vi "Read Acquisition Interface.vi"(8 "error in (no error)":errorcluster, 11 "Control_interface in":refnum<class "Control_interface.lvclass">) -> (0 "error out":errorcluster, 2 "Acquisition Interface":T1={"Sample Rate"=6000000000.0, "Clock mode"=enum."Internal", "Mode"=0, "Depth"=816000.0, "Segment Size"=816000.0, "Trigger Timeout"=-1.0, "Trigger Holdoff"=0.0, "Trigger Delay"=0.0} {"Segment Size" min=160.0 step=160.0; "Trigger Holdoff" min=0.0 step=160.0; "Trigger Delay" min=0.0 step=160.0; "Depth" min=160.0 step=160.0; "Mode" items=["Single", "Dual", "Quad", "Octal"]}, 3 "Control_interface out":refnum<class "Control_interface.lvclass">)   [LabVIEW 2015, in "Control_interface.lvclass"]
uses:
  Control_interface.lvclass
  Control_interface.lvclass/Control_interface.ctl
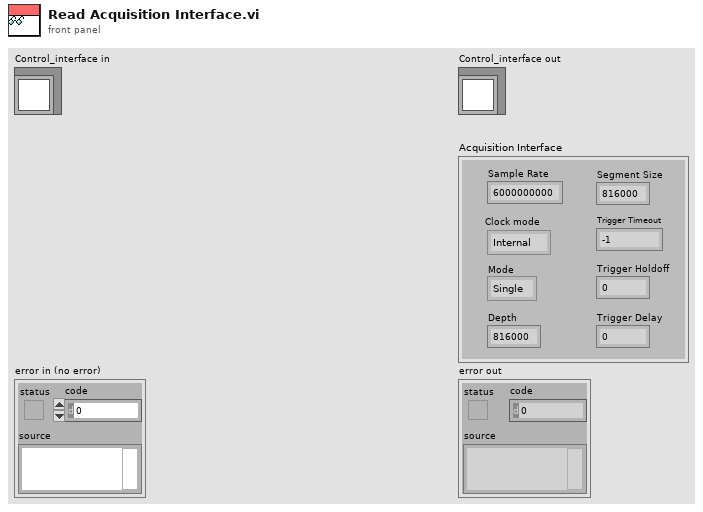
[diagram p1: front panel]
types:
  T1 = cluster{"Sample Rate":dbl, "Clock mode":enum16{"Internal", "External", "Reference"}, "Mode":u16, "Depth":dbl, "Segment Size":dbl, "Trigger Timeout":dbl, "Trigger Holdoff":dbl, "Trigger Delay":dbl}
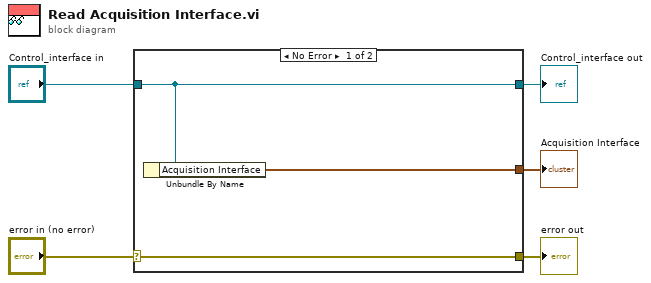
[diagram p0: block diagram]
diagram:
  n1 = case shown="No Error" "error in (no error)" {
    selector: "error in (no error)" -> [w8 w9]
    tunnel: [w8 w9] -> w4
    tunnel: [w7 w10] -> w2
    tunnel: "Control_interface in" -> [w7 w10]
    tunnel: [w6 _] -> w1
    frame No Error {
      n2 = Unbundle By Name(w7) -> ("Acquisition Interface"=w6:T1)
    }
    frame Error {
    }
  }
  "error out" <- w4
  "Control_interface out" <- w2
  "Acquisition Interface" <- w1
